vi "Calculate_dR_101-11-1.vi"(1 "[IN] Index of \"101\"\nDisplacement":i32, 2 "[IN] Subtrack":dbl[](array[numeric])) -> (0 "[OUT] Displacement average":dbl)   [LabVIEW 2013]
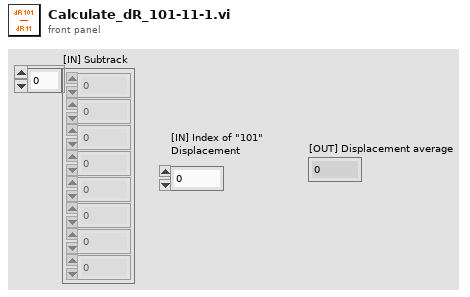
[diagram p1: front panel]
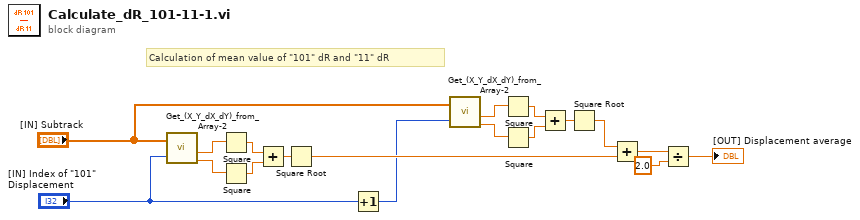
[diagram p0: block diagram]
diagram:
  # "Calculation of mean value of \"101\" dR and \"11\" dR"
  n1 = call "Get_(X_Y_dX_dY)_from_Array-2.vi"("(X,Y,dX,dY)"="[IN] Subtrack", "Index of Displacement"="[IN] Index of \"101\"\nDisplacement") -> ("dX"=w15:dbl, "dY"=w14:dbl)  [unwired: 2 out]
  n2 = Square(x=w15) -> (x^2=w18:dbl)
  n3 = Square(x=w14) -> (x^2=w17:dbl)
  n4 = Add(x=w18, y=w17) -> (x+y=w16:dbl)
  n5 = Square Root(x=w16) -> (sqrt(x)=w7:dbl)
  n6 = Increment(x="[IN] Index of \"101\"\nDisplacement") -> (x+1=w5:i32)
  n7 = call "Get_(X_Y_dX_dY)_from_Array-2.vi"("(X,Y,dX,dY)"="[IN] Subtrack", "Index of Displacement"=w5) -> ("dX"=w10:dbl, "dY"=w9:dbl)  [unwired: 2 out]
  n8 = Square(x=w10) -> (x^2=w13:dbl)
  n9 = Square(x=w9) -> (x^2=w12:dbl)
  n10 = Add(x=w13, y=w12) -> (x+y=w11:dbl)
  n11 = Square Root(x=w11) -> (sqrt(x)=w8:dbl)
  n12 = Add(x=w8, y=w7) -> (x+y=w3:dbl)
  n13 = Divide(x=w3, y=2.0) -> (x/y=→"[OUT] Displacement average":dbl)
